vi "load_clz_data.vi"(7 "matched set":set{cluster{"CLZ id":i32, "CV id":i32}}(c389), 8 "error in (no error)":errorcluster, 10 "report path":path=path "D:/Comics/data/Complete_CLZ_collection.csv", 11 "Volumes in":refnum<class "Volumes.lvclass">) -> (0 "error out":errorcluster, 3 "Volumes out":refnum<class "Volumes.lvclass">)   [LabVIEW 2024, in "CLZ_to_ComicVine.lvlib" / "Volumes.lvclass"]
uses:
  Volumes.lvclass
  typedefs/volume--cluster.ctl
  Volumes.lvclass/Volumes.ctl
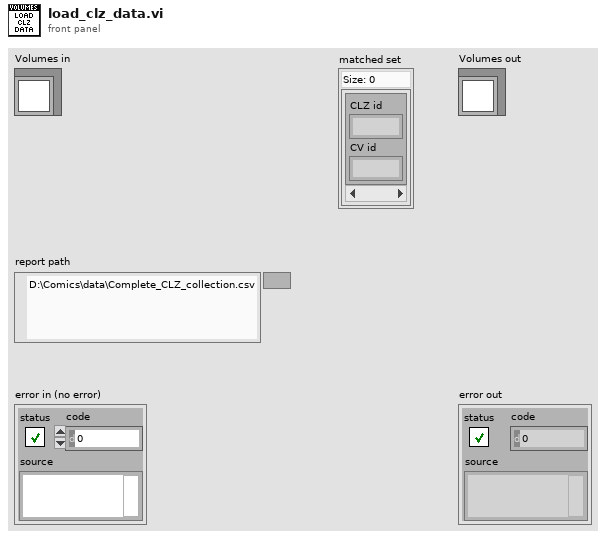
[diagram p1: front panel]
types:
  T1 = typedef "CLZ_to_ComicVine.lvlib/Volumes.lvclass/volume--cluster.ctl" = cluster{"id":i32, "name":string, "issue set":set{string}, "matched":bool}
  T2 = typedef "CLZ_to_ComicVine.lvlib/CLZ_comic.ctl" = cluster{"Series":string, "Core SeriesID":i32, "Core ComicID":i32, "Issue":string, "Variant":string}
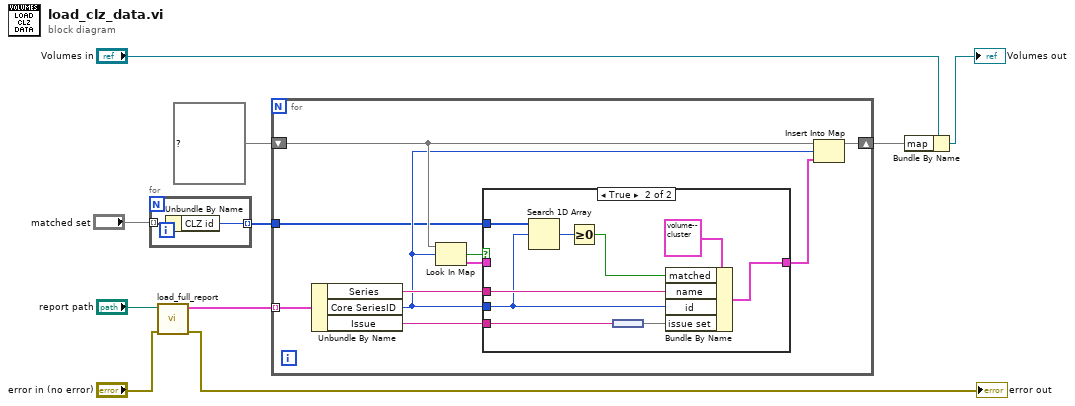
[diagram p0: block diagram]
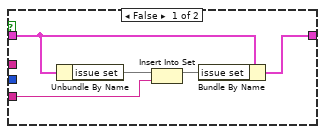
[diagram p2: hidden frame]
diagram:
  n1 = for {
    tunnel: "matched set" -> [w12] mode=indexing
    tunnel: [w11] -> w1 mode=indexing
    n2 = Unbundle By Name(w12) -> ("CLZ id"=w11:i32)
  }
  n3 = call "load_full_report.vi"("error in (no error)"="error in (no error)", "report path"="report path") -> ("error out"=→"error out":errorcluster, "clz_comics"=w7:T2[])  [unwired: 8 in]
  n4 = for {
    tunnel: w7 -> [w22] mode=indexing
    shift-right: [w16] -> w3
    shift-left: map{i32, T1} {} ("map") -> [w19]
    tunnel: w1 -> [w13]
    n5 = Unbundle By Name(w22) -> ("Series"=w20:string, "Core SeriesID"=w18:i32, "Issue"=w14:string)
    n6 = Look In Map(map=w19, key=w18) -> (key not found?=w21:bool, value=w15:T1)  [unwired: 1 in]
    n7 = case shown="True" w21 {
      tunnel: w20 -> [_ w36]
      tunnel: w18 -> [_ w30]
      tunnel: [w24 w35] -> w17
      tunnel: w15 -> [w27 _]
      tunnel: w14 -> [w23 w34]
      tunnel: w13 -> [_ w31]
      frame False {
        n8 = Unbundle By Name(w27) -> ("issue set"=w26:set{string})
        n9 = Insert Into Set(10:w23, 11:w26) -> (3:w25:set{string})  [unwired: 1 out]
        n10 = Bundle By Name(cluster=w27, "issue set"=w25) -> (w24:T1)
      }
      frame True {
        n11 = Search 1D Array(1D array=w31, element=w30) -> (index of element=w29:i32)  [unwired: 1 in]
        n12 = Greater Or Equal To 0?(x=w29) -> (x >= 0?=w28:bool)
        n13 = node(w34) -> (w33:set{string})
        n14 = Bundle By Name(cluster=T1 {"id"=0, "name"="", "issue set"={}, "matched"=FALSE} ("volume"), "matched"=w28, "name"=w36, "id"=w30, "issue set"=w33) -> (w35:T1)
      }
    }
    n15 = Insert Into Map(map in=w19, key=w18, value=w17) -> (map out=w16:map{i32, T1})  [unwired: 2 out]
  }
  n16 = Bundle By Name(cluster="Volumes in", "map"=w3) -> (→"Volumes out":refnum<class "Volumes.lvclass">)
